vi "Check position str.vi"(7 "°/step":dbl[](array[numeric]) format="%#_13g", 8 "error in (no error)":errorcluster, 9 "Motor params":T1={"Action"=2, "Direction motor 1"=1, "Direction motor 2"=1, "Steps motor 1"=100, "Steps motor 2"=100, "Step style motor 1"=1, "Step style motor 2"=1} {"Step style motor 2" items=["", "Single", "Double", "Interleave", "Microstep"]; "Step style motor 1" items=["", "Single", "Double", "Interleave", "Microstep"]; "Direction motor 2" items=["", "Forward", "Backward"]; "Direction motor 1" items=["", "Forward", "Backward"]; "Action" items=["", "Initialize", "Move"]}, 10 "Positions":dbl[](array[numeric]), 11 "Recibo de Datos":string) -> (0 "error out":errorcluster, 3 "Positions out":dbl[](array[numeric]))   [LabVIEW 2025, in "Control de MaP.lvlib"]
uses:
  Control de MaP.lvlib
  Controls/Move motor parameters--cluster.ctl
  Controls/Motor direction.ctl
  Controls/Step style.ctl
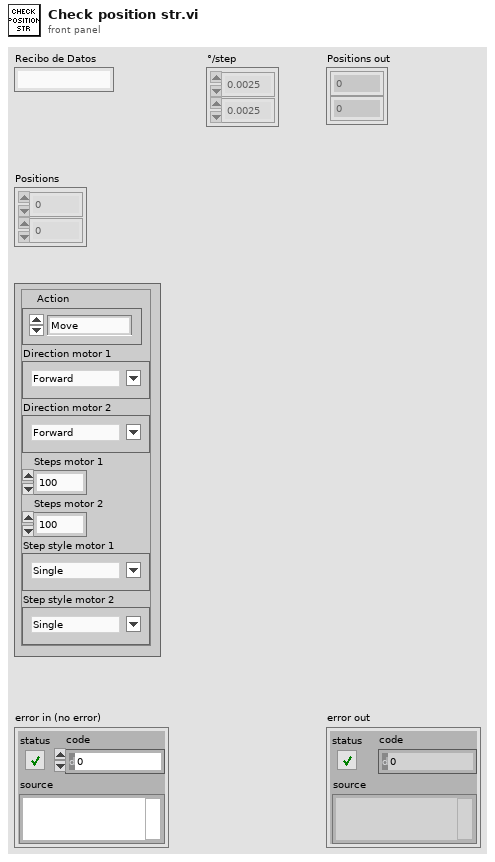
[diagram p1: front panel]
types:
  T1 = typedef "Control de MaP.lvlib/Move motor parameters--cluster.ctl" = cluster{"Action":u8, "Direction motor 1":T2, "Direction motor 2":T2, "Steps motor 1":u16, "Steps motor 2":u16, "Step style motor 1":T3, "Step style motor 2":T3}
  T2 = typedef "Control de MaP.lvlib/Motor direction.ctl" = u8
  T3 = typedef "Control de MaP.lvlib/Step style.ctl" = u8
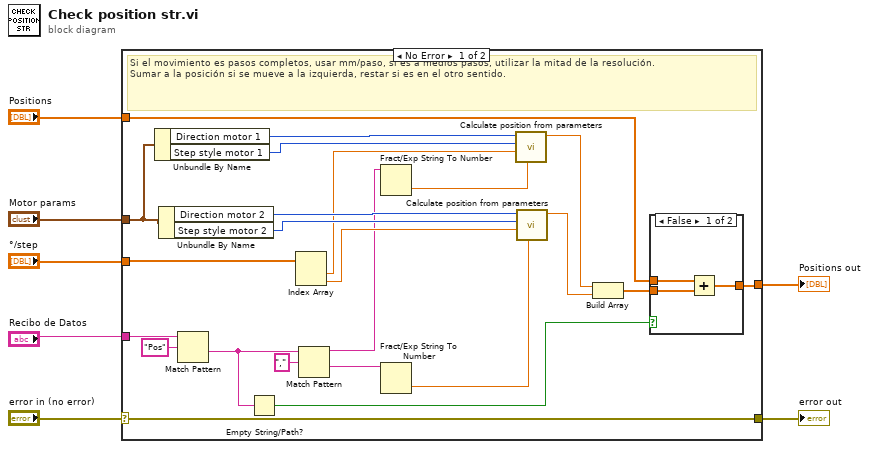
[diagram p0: block diagram]
diagram:
  n1 = case shown="No Error" "error in (no error)" {
    selector: "error in (no error)" -> [w28 w36]
    tunnel: [w25 w35] -> w7
    tunnel: "Positions" -> [w24 w35]
    tunnel: "Recibo de Datos" -> [w29 _]
    tunnel: [w28 w36] -> w3
    tunnel: "Motor params" -> [w22 _]
    tunnel: "°/step" -> [w19 _]
    frame No Error {
      # "Si el movimiento es pasos completos, usar mm/paso, si es a medios pasos, utilizar la mitad de la resolución.\nSumar a la posición si se mueve a la izquierda, restar si es en el otro sentido."
      n2 = Unbundle By Name(w22) -> ("Direction motor 1"=w26:T2, "Step style motor 1"=w27:T3)
      n3 = Unbundle By Name(w22) -> ("Direction motor 2"=w20:T2, "Step style motor 2"=w21:T3)
      n4 = Match Pattern(string=w29, regular expression="Pos") -> (after substring=w12:string)  [unwired: 1 in, 3 out]
      n5 = Empty String/Path?(string/path=w12) -> (empty?=w23:bool)
      n6 = Index Array(array=w19) -> (element #1=w18:dbl, element #2=w17:dbl)  [unwired: 2 in]
      n7 = Match Pattern(string=w12, regular expression=",") -> (before substring=w8:string, after substring=w10:string)  [unwired: 1 in, 2 out]
      n8 = Fract/Exp String To Number(string=w8) -> (number=w13:dbl)  [unwired: 3 in, 1 out]
      n9 = Fract/Exp String To Number(string=w10) -> (number=w9:dbl)  [unwired: 3 in, 1 out]
      n10 = call "Calculate position from parameters.vi"("Current step"=w13, "°/step"=w18, "Step style motor"=w27, "Motor direction"=w26) -> ("Position adjustment"=w15:dbl)  [unwired: 6 in, 1 out]
      n11 = call "Calculate position from parameters.vi"("Current step"=w9, "°/step"=w17, "Step style motor"=w21, "Motor direction"=w20) -> ("Position adjustment"=w14:dbl)  [unwired: 6 in, 1 out]
      n12 = Build Array(w15, w14) -> (w16:dbl[])
      n13 = case shown="False" w23 {
        tunnel: [w33 w34] -> w25
        tunnel: w16 -> [w32 _]
        tunnel: w24 -> [w31 w34]
        frame False {
          n14 = Add(x=w31, y=w32) -> (x+y=w33:dbl[])
        }
        frame True {
        }
      }
    }
    frame Error {
    }
  }
  "Positions out" <- w7
  "error out" <- w3
